vi "Memory.Pointer.Internal.Allocate.vi"(8 "error in (no error)":errorcluster, 10 "size":u64 format="%08x bytes", 11 "pointer in":refnum<class "Memory.Pointer.Internal.lvclass">) -> (0 "error out":errorcluster, 3 "pointer out":refnum<class "Memory.Pointer.Internal.lvclass">)   [LabVIEW 2016, in "Memory.lvlib" / "Memory.Pointer.Internal.lvclass"]
uses:
  Memory.Pointer.Internal.lvclass
  C:/Git/SourceTree/DSF/Source/Submodules/Memory/Source/Classes/Pointer/Memory.Pointer.lvclass
  Pointer/Memory.Pointer.lvclass/Memory.Pointer.ctl
  Pointer/Memory.Pointer.lvclass
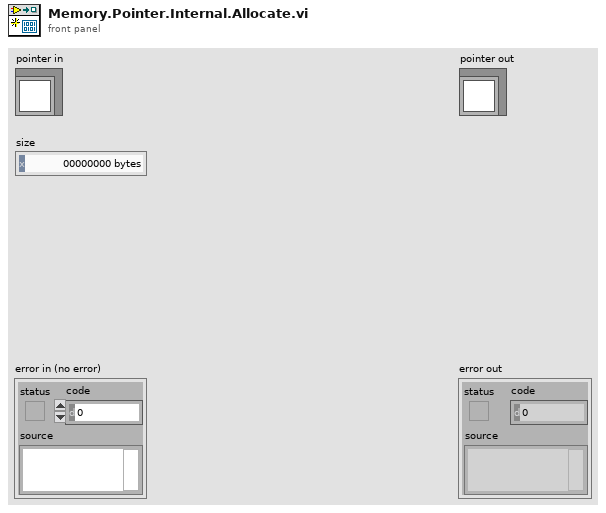
[diagram p1: front panel]
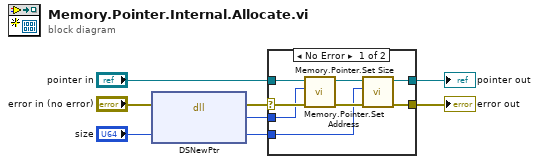
[diagram p0: block diagram]
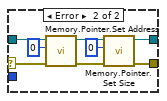
[diagram p2: hidden frame]
diagram:
  n1 = dll-call lib="LabVIEW" fn="DSNewPtr"(error in="error in (no error)", "size"="size") -> (error out=w6:errorcluster, "pointer"=w8:u64, "size"=w7:u64)  [unwired: 2 in, 1 out]
  n2 = case shown="No Error" w6 {
    selector: w6 -> [w15 w17]
    tunnel: "pointer in" -> [w16 w20]
    tunnel: w8 -> [w14 _]
    tunnel: [w11 w19] -> w5
    tunnel: w7 -> [w9 _]
    tunnel: [w10 w18] -> w3
    frame No Error {
      n3 = call "Memory.Pointer.Set Address.vi"("error in (no error)"=w15, "address"=w14, "Pointer in"=w16) -> ("error out"=w12:errorcluster, "Pointer out"=w13:refnum<class "Memory.Pointer.Internal.lvclass">)  [unwired: 7 in]
      n4 = call "Memory.Pointer.Set Size.vi"("error in (no error)"=w12, "size"=w9, "Pointer in"=w13) -> ("error out"=w10:errorcluster, "Pointer out"=w11:refnum<class "Memory.Pointer.Internal.lvclass">)  [unwired: 7 in]
    }
    frame Error {
      n5 = call "Memory.Pointer.Set Address.vi"("error in (no error)"=w17, "address"=u64 0, "Pointer in"=w20) -> ("error out"=w21:errorcluster, "Pointer out"=w22:refnum<class "Memory.Pointer.Internal.lvclass">)  [unwired: 7 in]
      n6 = call "Memory.Pointer.Set Size.vi"("error in (no error)"=w21, "size"=u64 0, "Pointer in"=w22) -> ("error out"=w18:errorcluster, "Pointer out"=w19:refnum<class "Memory.Pointer.Internal.lvclass">)  [unwired: 7 in]
    }
  }
  "error out" <- w3
  "pointer out" <- w5
